vi "Begin.vi"(8 "error in":errorcluster) -> (0 "error out":errorcluster)   [LabVIEW 2015]
doc: "Called before other user functions, this VI is expected to open initial I/O refnums, load in file data, and do all program initialization. Notice that the <B>error out</B> terminal is simply used for data flow. Wiring it to other structures or subVIs ensures that this VI runs first."
uses:
  <vilib>/Rock Robotics/WPI/DriverStation/WPI_DriverStationRobotMode2.ctl
  <vilib>/Rock Robotics/WPI/SafetyOutput/WPI_SafetyOutputConfigMenu.ctl
  <vilib>/Rock Robotics/WPI/Joystick/WPI_JoystickDeviceEnum.ctl
  <vilib>/Rock Robotics/WPI/Solenoid/WPI_SolenoidChannel.ctl
  <vilib>/Rock Robotics/SystemInterfaces/AI/FPGA_AIChannel.ctl
  <vilib>/Rock Robotics/SystemInterfaces/DIO/FPGA_DIOChannel.ctl
  <vilib>/Rock Robotics/WPI/Encoder/WPI_EncoderType.ctl
  <vilib>/Rock Robotics/SystemInterfaces/DIO/FPGA_DIOPWMChannel.ctl
  Robot Global Data.vi
  <vilib>/Rock Robotics/Network Tables/NT Write String Array.vi
  <vilib>/Rock Robotics/WPI/RobotDrive/WPI_RobotDriveOpen4MotorWithCANTalonSRX.vi
  <vilib>/Rock Robotics/WPI/MotorControl/WPI_MotorControlOpenCANTalonSRX.vi
  <vilib>/Rock Robotics/WPI/Utilities/WPI_GetSetVariantRefNum.vi
  <vilib>/Rock Robotics/WPI/Solenoid/WPI_SolenoidOpenSingle.vi
  <vilib>/Rock Robotics/WPI/Counter/WPI_CounterDigitalInputToDigitalSource.vi
  <vilib>/Rock Robotics/WPI/Solenoid/WPI_SolenoidOpenDouble.vi
  <vilib>/Rock Robotics/WPI/CAN/TalonSRX/WPI_CANTalonSRX_APIControlMode.ctl
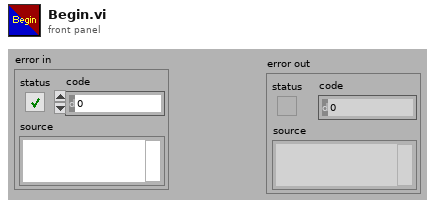
[diagram p1: front panel]
types:
  T1 = typedef "FPGA_DIOPWMChannel.ctl" = enum8{"PWM 0", "PWM 1", "PWM 2", "PWM 3", "PWM 4", "PWM 5", "PWM 6", "PWM 7", "PWM 8", "PWM 9", "PWM MXP 0", "PWM MXP 1", "PWM MXP 2", "PWM MXP 3", "PWM MXP 4", "PWM MXP 5", "PWM MXP 6", "PWM MXP 7", "PWM MXP 8", "PWM MXP 9", "Invalid"}
  T2 = typedef "WPI_SolenoidChannel.ctl" = enum8{"Solenoid 0", "Solenoid 1", "Solenoid 2", "Solenoid 3", "Solenoid 4", "Solenoid 5", "Solenoid 6", "Solenoid 7", "Invalid"}
  T3 = typedef "WPI_EncoderType.ctl" = enum16{"1x", "2x", "4x"}
  T4 = typedef "FPGA_DIOChannel.ctl" = enum8{"DIO 0", "DIO 1", "DIO 2", "DIO 3", "DIO 4", "DIO 5", "DIO 6", "DIO 7", "DIO 8", "DIO 9", "DIO MXP 0", "DIO MXP 1", "DIO MXP 2", "DIO MXP 3", "DIO MXP 4", "DIO MXP 5", "DIO MXP 6", "DIO MXP 7", "DIO MXP 8", "DIO MXP 9", "DIO MXP 10", "DIO MXP 11", "DIO MXP 12", "DIO MXP 13", "DIO MXP 14", "DIO MXP 15", "Invalid"}
  T5 = typedef "FPGA_AIChannel.ctl" = enum8{"AI 0", "AI 1", "AI 2", "AI 3", "AI MXP 0", "AI MXP 1", "AI MXP 2", "AI MXP 3", "Invalid"}
  T6 = typedef "WPI_JoystickDeviceEnum.ctl" = enum16{"USB 0", "USB 1", "USB 2", "USB 3", "USB 4", "USB 5"}
  T7 = typedef "WPI_SafetyOutputConfigMenu.ctl" = enum16{"Enable", "Disable"}
  T8 = typedef "WPI_DriverStationRobotMode2.ctl" = enum16{"Autonomous Disabled", "Autonomous Enabled", "Teleop Disabled", "Teleop Enabled", "Disconnected", "Finish", "Test Disabled", "Test Enabled", "Emergency Stopped"}
  T9 = typedef "WPI_CANTalonSRX_APIControlMode.ctl" = enum8{"Percent VBus", "Speed", "Position", "Slave", "Unchanged / Invalid", "Voltage Compensation", "Current", "Motion Profile"}
  T10 = typedef "WPI_MotorControlDeviceRef.ctl" = cluster{"DeviceStatus":errorcluster, "Type":T11, "PWM":cluster{"PWM Channel":T1, "DeadBand":T12}, "CAN":cluster{"Device Number":u8, "Control Mode":T13, "Semaphore":T14, "Max Vout":dbl, "TalonSRX Control Mode":T9}, "Invert":bool}
  T11 = typedef "WPI_MotorControlType.ctl" = enum16{"PWM", "CAN", "CANTalonSRX"}
  T12 = typedef "WPI_PWMDeadband.ctl" = cluster{"Name":string, "maxPositivePwm":i32, "minPositivePwm":i32, "centerPwm":i32, "maxNegativePwm":i32, "minNegativePwm":i32, "angularRange":u16}
  T13 = typedef "WPI_CANJaguar_ControlMode.ctl" = enum8{"Percent VBus", "Current", "Speed", "Position", "Voltage"}
  T14 = typedef "Semaphore RefNum" = refnum<k1>
  T15 = typedef "WPI_CompressorDevRef.ctl" = cluster{"DevStatus":errorcluster, "Pneumatics Control Module":u8}
  T16 = typedef "WPI_RobotDriveDevRef.ctl" = cluster{"DevStatus":errorcluster, "Motors[]":T10[], "Square Inputs":bool, "Max Output":dbl}
  T17 = typedef "WPI_AnalogChannelDevRef.ctl" = cluster{"DevStatus":errorcluster, "Analog Channel":T5}
  T18 = typedef "WPI_DigitalInputDevRef.ctl" = cluster{"DevStatus":errorcluster, "DIO Channel":T4}
  T19 = typedef "WPI_JoystickDevRef.ctl" = cluster{"Device":T6}
  T20 = typedef "FPGA_CounterEncoderSourceConvertionLVSourceType.ctl" = cluster{"DevStatus":errorcluster, "AnalogTriggerMode?":bool, "DigitalMode":cluster{"DIO Channel":T21}, "AnalogTriggerMode":cluster{"AnalogTriggerIndex":T22, "OutputType":T23}}
  T21 = typedef "FPGA_DIODigitalSourceChannel.ctl" = enum8{"DIO 0", "DIO 1", "DIO 2", "DIO 3", "DIO 4", "DIO 5", "DIO 6", "DIO 7", "DIO 8", "DIO 9", "DIO MXP 0", "DIO MXP 1", "DIO MXP 2", "DIO MXP 3", "DIO MXP 4", "DIO MXP 5", "DIO MXP 6", "DIO MXP 7", "DIO MXP 8", "DIO MXP 9", "DIO MXP 10", "DIO MXP 11", "DIO MXP 12", "DIO MXP 13", "DIO MXP 14", "DIO MXP 15", "Disabled"}
  T22 = typedef "FPGA_AnalogTriggerIndex.ctl" = enum8{"Trig 0", "Trig 1", "Trig 2", "Trig 3", "Trig 4", "Trig 5", "Trig 6", "Trig 7", "Invalid"}
  T23 = typedef "FPGA_AnalogTriggerOutType.ctl" = enum16{"InWindow", "TriggerState", "Rising", "Falling"}
  T24 = typedef "WPI_EncoderDevRef.ctl" = cluster{"DevStatus":errorcluster, "EncoderIndex":T25, "CounterIndex":T26, "DistancePerCount":dbl, "Decoding Type":T3}
  T25 = typedef "FPGA_EncoderIdx.ctl" = enum8{"Enc 0", "Enc 1", "Enc 2", "Enc 3", "Enc 4", "Enc 5", "Enc 6", "Enc 7", "Invalid"}
  T26 = typedef "FPGA_CounterCtrSystemIndex.ctl" = enum8{"Ctr 0", "Ctr 1", "Ctr 2", "Ctr 3", "Ctr 4", "Ctr 5", "Ctr 6", "Ctr 7", "Invalid"}
  T27 = typedef "WPI_SolenoidDevRef.ctl" = cluster{"DevStatus":errorcluster, "Pneumatics Control Module":u8, "Forward Solenoid Channel":T2, "Reverse Solenoid Channel":T2}
  T28 = typedef "WPI_ServoDeviceRef.ctl" = cluster{"DeviceStatus":errorcluster, "PWM Channel":T1, "DeadBand":T12}
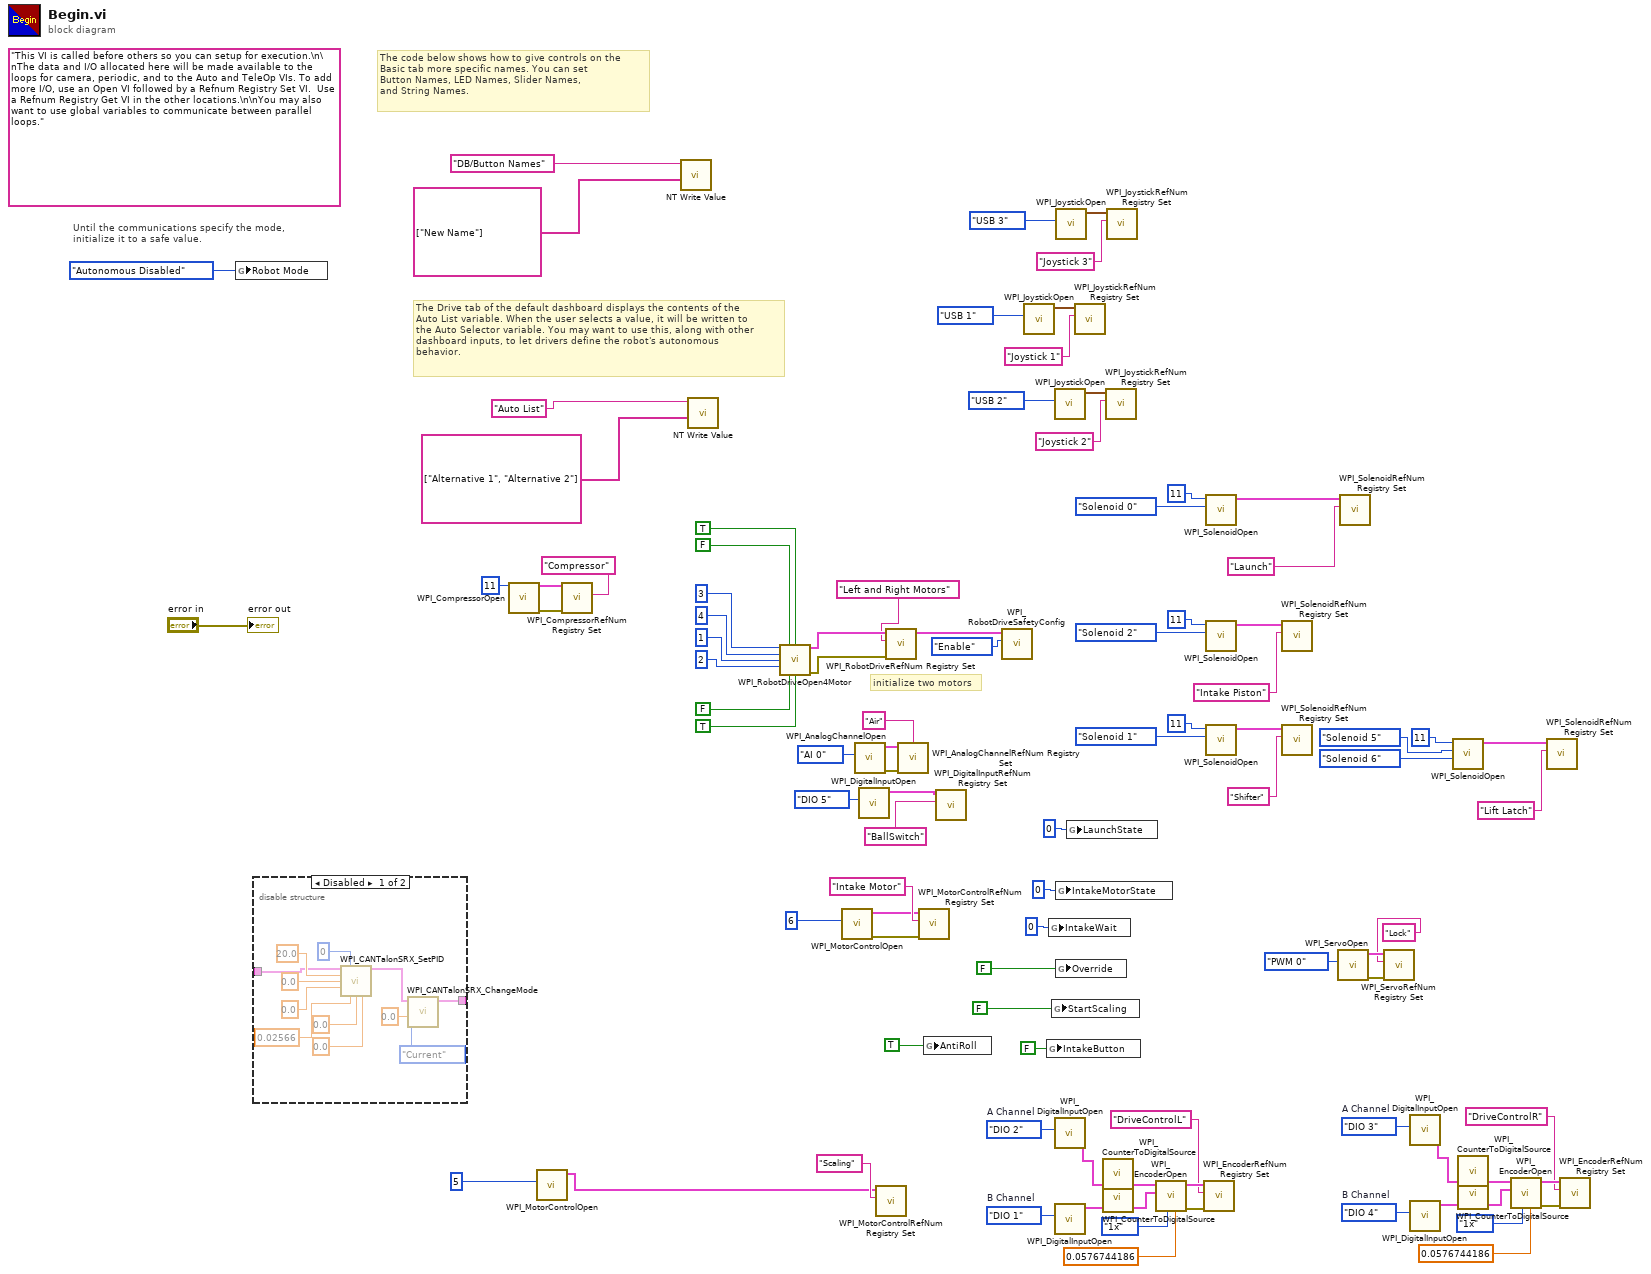
[diagram p0: block diagram]
diagram:
  w19 = FPGA_DIOChannel."DIO 4"  # B Channel
  w18 = FPGA_DIOChannel."DIO 3"  # A Channel
  w30 = FPGA_DIOChannel."DIO 1"  # B Channel
  w29 = FPGA_DIOChannel."DIO 2"  # A Channel
  (unwired) "This VI is called before others so you can setup for execution.\n\nThe data and I/O allocated here will be made available to the loops for camera, periodic, and to the Auto and TeleOp VIs. To add more I/O, use an Open VI followed by a Refnum Registry Set VI.  Use a Refnum Registry Get VI in the other locations.\n\nYou may also want to use global variables to communicate between parallel loops."
  # "initialize two motors"
  # "The Drive tab of the default dashboard displays the contents of the\nAuto List variable. When the user selects a value, it will be written to\nthe Auto Selector variable. You may want to use this, along with other\ndashboard inputs, to let drivers define the robot's autonomous\nbehavior."
  # "The code below shows how to give controls on the\nBasic tab more specific names. You can set\nButton Names, LED Names, Slider Names,\nand String Names."
  # "Until the communications specify the mode,\ninitialize it to a safe value."
  n1 = global write "Robot Global Data.vi" "Robot Mode"(WPI_DriverStationRobotMode2."Autonomous Disabled" ("Robot Mode")) -> ()
  n2 = disable-structure shown="Disabled" {
    disable-tunnel: _ -> [w101 _]
    disable-tunnel: [w97 _] -> _
    frame Disabled {
      n3 = call <vilib>:"WPI_CANTalonSRX_SetPID.vi"("CAN Talon SRX Ref"=w101, "Parameter Slot"=u8 0, "P"=20.0, "I"=0.0, "D"=0.0, "F"=0.02566, "I Zone"=0.0, "Ramp Rate"=0.0) -> ("CAN Talon SRX Ref"=w100:T10)  [unwired: 6 in, 1 out]
      n4 = call <vilib>:"WPI_CANTalonSRX_ChangeMode.vi"("Output"=0.0, "Control Mode"=WPI_CANTalonSRX_APIControlMode."Current", "CAN Talon SRX Ref"=w100) -> ("CAN Talon SRX Ref"=w97:T10)  [unwired: 7 in, 1 out]
    }
    frame Enabled {
    }
  }
  n5 = call <vilib>:"WPI_CompressorOpen.vi"("Pneumatics Control Module (0)"=u8 11) -> ("CompressorDevRef"=w52:T15, "error out"=w53:errorcluster)  [unwired: 13 in]
  n6 = call-poly <vilib>:"WPI_MotorControlOpen.vi"("Device Number"=u8 5) -> ("MotorControlDeviceRef"=w2:T10)  [unwired: 9 in, 1 out]
  n7 = call <vilib>:"WPI_CompressorRefNum Registry Set.vi"("error in (no error)"=w53, "refnum name"="Compressor", "CompressorDevRef"=w52) -> ()  [unwired: 7 in, 2 out]
  n8 = call-poly <vilib>:"NT Write Value.vi"("String Array"=string[] ["New Name"], "Name"="DB/Button Names") -> ()  [unwired: 9 in, 1 out]
  n9 = call-poly <vilib>:"NT Write Value.vi"("String Array"=string[] ["Alternative 1", "Alternative 2"], "Name"="Auto List") -> ()  [unwired: 9 in, 1 out]
  n10 = call-poly <vilib>:"WPI_RobotDriveOpen4Motor.vi"("Rear Left Motor"=u8 3, "Rear Left Motor Inverted"=FALSE, "Rear Right Motor Inverted"=TRUE, "Rear Right Motor"=u8 4, "Front Left Motor"=u8 1, "Front Right Motor"=u8 2, "Front Left Motor Inverted"=FALSE, "Front Right Motor Inverted"=TRUE) -> ("RobotDriveDevRef"=w90:T16, "error out"=w88:errorcluster)  [unwired: 6 in]
  n11 = call-poly <vilib>:"WPI_MotorControlOpen.vi"("Device Number"=u8 6) -> ("error out"=w76:errorcluster, "MotorControlDeviceRef"=w3:T10)  [unwired: 9 in]
  n12 = call <vilib>:"WPI_AnalogChannelOpen.vi"("Analog Channel"=FPGA_AIChannel."AI 0") -> ("error out"=w49:errorcluster, "AIDeviceRef"=w48:T17)  [unwired: 9 in]
  n13 = call <vilib>:"WPI_DigitalInputOpen.vi"("DIO Channel"=FPGA_DIOChannel."DIO 5") -> ("DigitalInputDevRef"=w32:T18)  [unwired: 9 in, 1 out]
  n14 = call <vilib>:"WPI_MotorControlRefNum Registry Set.vi"("refnum name"="Scaling", "MotorControlDevRef"=w2) -> ()  [unwired: 8 in, 2 out]
  n15 = call <vilib>:"WPI_RobotDriveRefNum Registry Set.vi"("error in (no error)"=w88, "refnum name"="Left and Right Motors", "RobotDriveDevRef"=w90) -> ("RobotDriveDevRef"=w87:T16)  [unwired: 1 in, 7 out]
  n16 = call <vilib>:"WPI_AnalogChannelRefNum Registry Set.vi"("error in (no error)"=w49, "refnum name"="Air", "AIDeviceRef"=w48) -> ()  [unwired: 7 in, 2 out]
  n17 = call <vilib>:"WPI_MotorControlRefNum Registry Set.vi"("error in (no error)"=w76, "refnum name"="Intake Motor", "MotorControlDevRef"=w3) -> ()  [unwired: 7 in, 2 out]
  n18 = global write "Robot Global Data.vi" "AntiRoll"(TRUE ("IntakeButton")) -> ()
  n19 = call <vilib>:"WPI_DigitalInputRefNum Registry Set.vi"("refnum name"="BallSwitch", "DigitalInputDevRef"=w32) -> ()  [unwired: 8 in, 2 out]
  n20 = call <vilib>:"WPI_RobotDriveSafetyConfig.vi"("mode"=WPI_SafetyOutputConfigMenu."Enable", "RobotDriveDevRef"=w87) -> ()  [unwired: 8 in, 2 out]
  n21 = call <vilib>:"WPI_JoystickOpen.vi"("JoystickDevice"=WPI_JoystickDeviceEnum."USB 1") -> ("JoystickDevRef"=w71:T19)  [unwired: 10 in]
  n22 = global write "Robot Global Data.vi" "IntakeButton"(FALSE ("IntakeButton")) -> ()
  n23 = global write "Robot Global Data.vi" "IntakeWait"(u8 0 ("LaunchState")) -> ()
  n24 = global write "Robot Global Data.vi" "StartScaling"(FALSE ("Override")) -> ()
  n25 = call <vilib>:"WPI_JoystickOpen.vi"("JoystickDevice"=WPI_JoystickDeviceEnum."USB 2") -> ("JoystickDevRef"=w68:T19)  [unwired: 10 in]
  n26 = call <vilib>:"WPI_DigitalInputOpen.vi"("DIO Channel"=w29) -> ("DigitalInputDevRef"=w26:T18)  [unwired: 1 in, 9 out]
  n27 = call <vilib>:"WPI_DigitalInputOpen.vi"("DIO Channel"=w30) -> ("DigitalInputDevRef"=w27:T18)  [unwired: 1 in, 9 out]
  n28 = call <vilib>:"WPI_JoystickOpen.vi"("JoystickDevice"=WPI_JoystickDeviceEnum."USB 3") -> ("JoystickDevRef"=w65:T19)  [unwired: 10 in]
  n29 = global write "Robot Global Data.vi" "IntakeMotorState"(u8 0 ("LaunchState")) -> ()
  n30 = global write "Robot Global Data.vi" "Override"(FALSE ("Override")) -> ()
  n31 = global write "Robot Global Data.vi" "LaunchState"(u8 0 ("LaunchState")) -> ()
  n32 = call <vilib>:"WPI_JoystickRefNum Registry Set.vi"("refnum name"="Joystick 1", "JoystickDevRef"=w71) -> ()  [unwired: 8 in, 2 out]
  n33 = call-poly <vilib>:"WPI_CounterToDigitalSource.vi"("DigitalInputDevRef"=w26) -> ("Digital Source"=w25:T20)  [unwired: 6 out]
  n34 = call-poly <vilib>:"WPI_CounterToDigitalSource.vi"("DigitalInputDevRef"=w27) -> ("Digital Source"=w28:T20)  [unwired: 6 out]
  n35 = call <vilib>:"WPI_JoystickRefNum Registry Set.vi"("refnum name"="Joystick 2", "JoystickDevRef"=w68) -> ()  [unwired: 8 in, 2 out]
  n36 = call <vilib>:"WPI_JoystickRefNum Registry Set.vi"("refnum name"="Joystick 3", "JoystickDevRef"=w65) -> ()  [unwired: 8 in, 2 out]
  n37 = call <vilib>:"WPI_EncoderOpen.vi"("DistancePerCount"=0.0576744186, "Decoding Type"=WPI_EncoderType."1x", "BSource"=w28, "ASource"=w25) -> ("error out"=w23:errorcluster, "EncoderDevRef"=w24:T24)  [unwired: 4 in, 2 out]
  n38 = call <vilib>:"WPI_EncoderRefNum Registry Set.vi"("error in (no error)"=w23, "refnum name"="DriveControlL", "EncoderDevRef"=w24) -> ()  [unwired: 7 in, 2 out]
  n39 = call-poly <vilib>:"WPI_SolenoidOpen.vi"("Solenoid Channel"=WPI_SolenoidChannel."Solenoid 0" ("Forward Solenoid Channel"), "Pneumatics Control Module (0)"=u8 11) -> ("SolenoidDevRef"=w63:T27)  [unwired: 8 in, 1 out]
  n40 = call-poly <vilib>:"WPI_SolenoidOpen.vi"("Solenoid Channel"=WPI_SolenoidChannel."Solenoid 2", "Pneumatics Control Module (0)"=u8 11) -> ("SolenoidDevRef"=w59:T27)  [unwired: 8 in, 1 out]
  n41 = call-poly <vilib>:"WPI_SolenoidOpen.vi"("Solenoid Channel"=WPI_SolenoidChannel."Solenoid 1", "Pneumatics Control Module (0)"=u8 11) -> ("SolenoidDevRef"=w61:T27)  [unwired: 8 in, 1 out]
  n42 = call <vilib>:"WPI_SolenoidRefNum Registry Set.vi"("refnum name"="Intake Piston", "SolenoidDevRef"=w59) -> ()  [unwired: 8 in, 2 out]
  n43 = call <vilib>:"WPI_SolenoidRefNum Registry Set.vi"("refnum name"="Shifter", "SolenoidDevRef"=w61) -> ()  [unwired: 8 in, 2 out]
  n44 = call <vilib>:"WPI_ServoOpen.vi"("PWM Channel"=FPGA_DIOPWMChannel."PWM 0") -> ("error out"=w7:errorcluster, "ServoDeviceRef"=w6:T28)  [unwired: 9 in]
  n45 = call <vilib>:"WPI_SolenoidRefNum Registry Set.vi"("refnum name"="Launch", "SolenoidDevRef"=w63) -> ()  [unwired: 8 in, 2 out]
  n46 = call <vilib>:"WPI_ServoRefNum Registry Set.vi"("error in (no error)"=w7, "refnum name"="Lock", "ServoDeviceRef"=w6) -> ()  [unwired: 7 in, 2 out]
  n47 = call <vilib>:"WPI_DigitalInputOpen.vi"("DIO Channel"=w18) -> ("DigitalInputDevRef"=w15:T18)  [unwired: 1 in, 9 out]
  n48 = call <vilib>:"WPI_DigitalInputOpen.vi"("DIO Channel"=w19) -> ("DigitalInputDevRef"=w16:T18)  [unwired: 1 in, 9 out]
  n49 = call-poly <vilib>:"WPI_SolenoidOpen.vi"("Reverse Solenoid Channel"=WPI_SolenoidChannel."Solenoid 6", "Forward Solenoid Channel"=WPI_SolenoidChannel."Solenoid 5" ("Solenoid Channel"), "Pneumatics Control Module (0)"=u8 11) -> ("SolenoidDevRef"=w35:T27)  [unwired: 7 in, 1 out]
  n50 = call-poly <vilib>:"WPI_CounterToDigitalSource.vi"("DigitalInputDevRef"=w15) -> ("Digital Source"=w14:T20)  [unwired: 6 out]
  n51 = call-poly <vilib>:"WPI_CounterToDigitalSource.vi"("DigitalInputDevRef"=w16) -> ("Digital Source"=w17:T20)  [unwired: 6 out]
  n52 = call <vilib>:"WPI_EncoderOpen.vi"("DistancePerCount"=0.0576744186, "Decoding Type"=WPI_EncoderType."1x", "BSource"=w17, "ASource"=w14) -> ("error out"=w12:errorcluster, "EncoderDevRef"=w13:T24)  [unwired: 4 in, 2 out]
  n53 = call <vilib>:"WPI_SolenoidRefNum Registry Set.vi"("refnum name"="Lift Latch", "SolenoidDevRef"=w35) -> ()  [unwired: 8 in, 2 out]
  n54 = call <vilib>:"WPI_EncoderRefNum Registry Set.vi"("error in (no error)"=w12, "refnum name"="DriveControlR", "EncoderDevRef"=w13) -> ()  [unwired: 7 in, 2 out]
  "error out" <- "error in"
